vi "Pockels Cal-Check cal exists.vi"() -> (1 "-1 if Pockels cal does not exist":i32)   [LabVIEW 2013]
uses:
  Typedefs/Which path.ctl
  Globals/gl_Calibration globals.vi
  Program Files (x86)/National Instruments/LabVIEW 2013/user.lib/My Palettes.lib/Files & paths/Spreadsheet/Read From Spreadsheet File (string)-Mod.vi
panel:
  out "Wavelength value":dbl
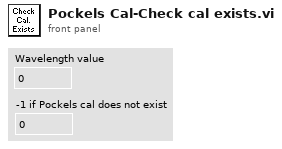
[diagram p1: front panel]
types:
  T1 = typedef "Which path.ctl" = enum16{"Configuration Files", "Calibration Files", "Images", "Setup.ini", "Loaded User profile.ini", "User's-Previous session.ini", "New user profile.ini", "Selected User profile.ini", "User profiles folder", "Power meter scaling.txt", "FOV Cal.ini"}
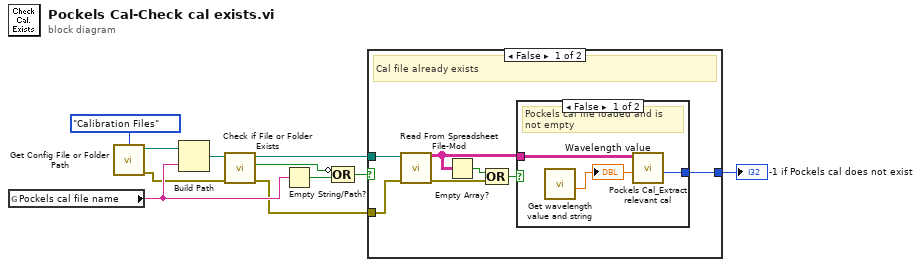
[diagram p0: block diagram]
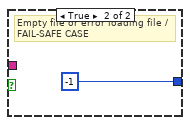
[diagram p2: hidden frame]
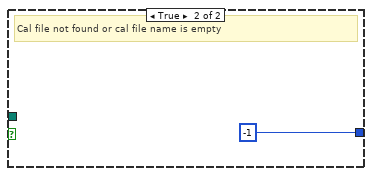
[diagram p3: hidden frame]
diagram:
  n1 = global read "gl_Calibration globals.vi" "Pockels cal file name"() -> (w8:string)
  n2 = call "Get Config File or Folder Path.vi"("Which file or folder?"=Which_path."Calibration Files" ("Which path?")) -> ("Error Out"=w2:errorcluster, "File Path"=w11:path)  [unwired: 8 in, 1 out]
  n3 = Build Path(base path=w11, name or relative path=w8) -> (appended path=w9:path)
  n4 = call <vilib>:"Check if File or Folder Exists.vi"("error in (no error)"=w2, "path"=w9) -> ("error out"=w3:errorcluster, "file or folder exists?"=w7:bool, "dup path"=w4:path)  [unwired: 7 in]
  n5 = Empty String/Path?(string/path=w8) -> (empty?=w6:bool)
  n6 = Compound Arithmetic op=OR(invert w7, w6) -> (w5:bool)
  n7 = case shown="False" w5 {
    tunnel: w4 -> [w16 _]
    tunnel: w3 -> [w15 _]
    tunnel: [w12 -1 ("Index of replacement")] -> w1
    frame False {
      # "Cal file already exists"
      n8 = call-poly "Read From Spreadsheet File-Mod.vi"("file path (dialog if empty)"=w16, "error in"=w15) -> ("all rows"=w13:string[][], "error out"=w14:errorcluster)  [unwired: 8 in, 4 out]
      n9 = Empty Array?(array=w13) -> (empty?=w17:bool)
      n10 = Compound Arithmetic op=OR(w17, w14) -> (w18:bool)
      n11 = case shown="False" w18 {
        tunnel: w13 -> [w21 _]
        tunnel: [w19 -1 ("Index of replacement")] -> w12
        frame False {
          # "Pockels cal file loaded and is not empty"
          n12 = call "Get wavelength value and string.vi"() -> ("Wavelength value"=w20:dbl)  [unwired: 9 in, 2 out]
          "Wavelength value" <- w20
          n13 = call "Pockels Cal_Extract relevant cal.vi"("Wavelength value"=w20, "Loaded table"=w21) -> ("Index of replacement"=w19:i32)  [unwired: 6 in, 3 out]
        }
        frame True {
          # "Empty file or error loading file / FAIL-SAFE CASE"
        }
      }
    }
    frame True {
      # "Cal file not found or cal file name is empty"
    }
  }
  "-1 if Pockels cal does not exist" <- w1
